vi "lookup_node_successors_by_id.vi"(10 "node_id":refnum<class "ID.lvclass">, 11 "self":refnum<class "DiGraph.lvclass">) -> (1 "successor_ids":set{refnum<class "ID.lvclass">}(c389), 2 "node not found?":bool)   [LabVIEW 2020, in "graph.lvlib" / "DiGraph.lvclass"]
uses:
  DiGraph.lvclass
  ID/ID.lvclass
  DiGraph.lvclass/DiGraph.ctl
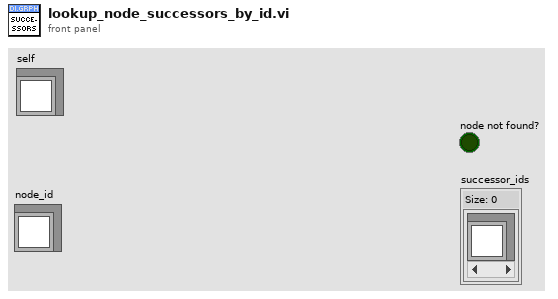
[diagram p1: front panel]
types:
  T1 = map{refnum<class "ID.lvclass">, set{refnum<class "ID.lvclass">}}
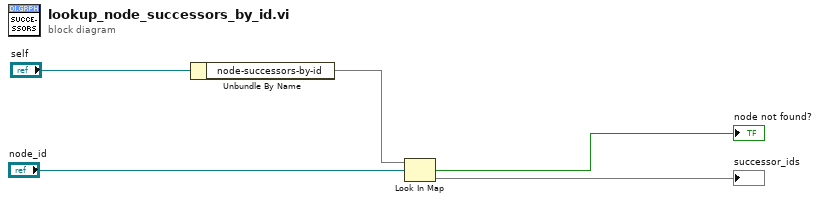
[diagram p0: block diagram]
diagram:
  n1 = Unbundle By Name("self") -> ("node-successors-by-id"=w2:T1)
  n2 = Look In Map(map=w2, key="node_id") -> (key not found?=→"node not found?":bool, value=→"successor_ids":set{refnum<class "ID.lvclass">})  [unwired: 1 in]
